vi "acq_and_background.vi"(9 "Acquisition Parameters":refnum<vi>[](array[refnum]), 11 "LightField Automation in":refnum<class "LightField Automation.lvclass">) -> (1 "DAQmx":dbl[][](array[numeric]), 2 "CCD":dbl[](array[numeric]), 3 "LightField Automation out":refnum<class "LightField Automation.lvclass">)   [LabVIEW 2015]
uses:
  lightfield-automation-labview/LightField Automation.lvclass
panel:
  out "Increment piezo":dbl
  out "Piezo":dbl
  out "DAQmx Task Shutter":refnum<k21>
  out "Shutter":string
  out "Background":string
  out "Accumulations":i32
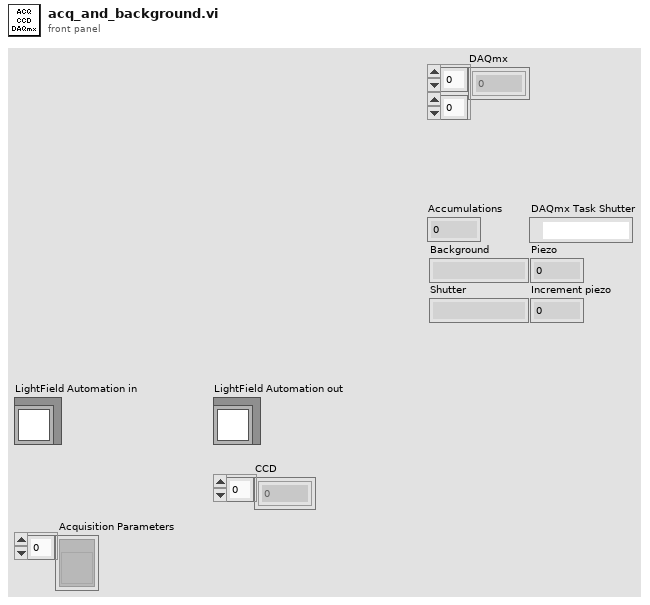
[diagram p1: front panel]
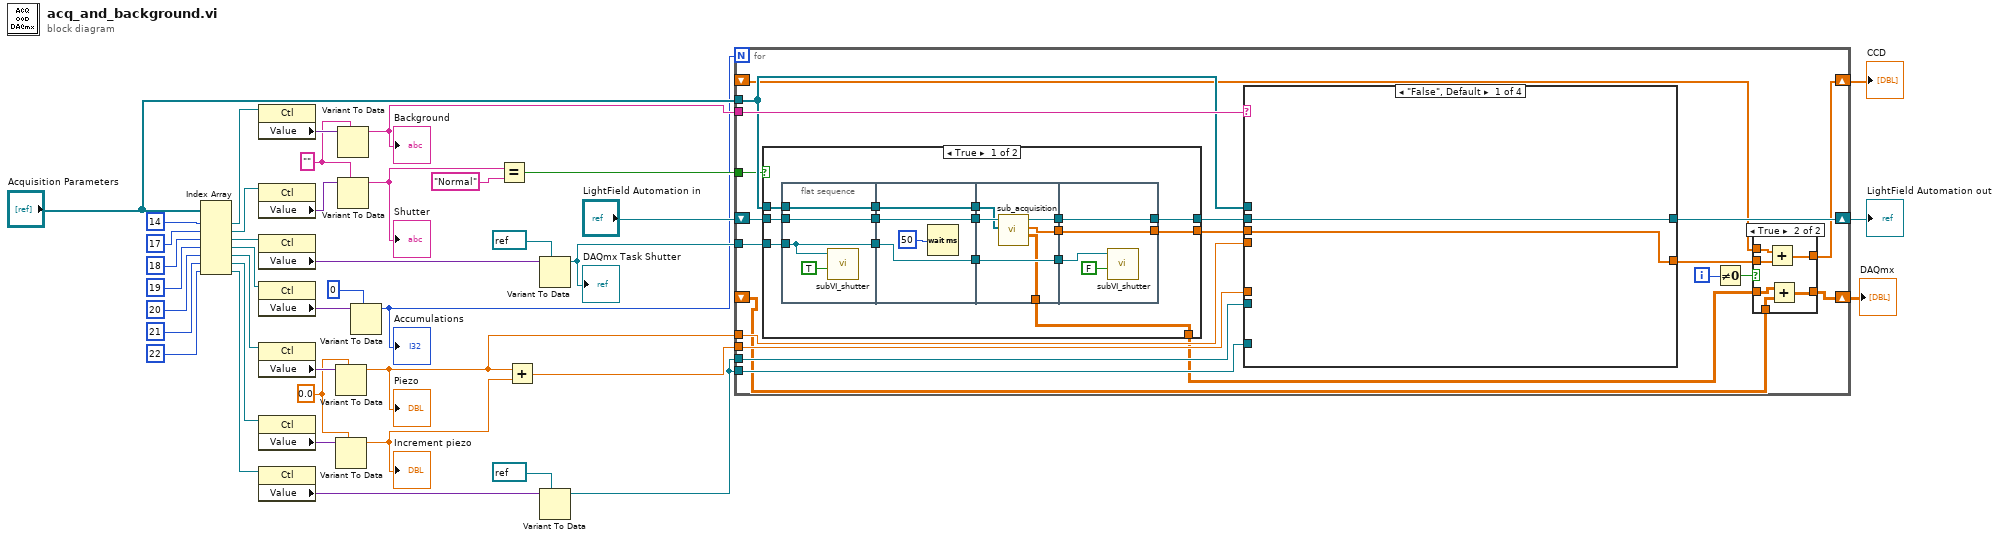
[diagram p0: block diagram]
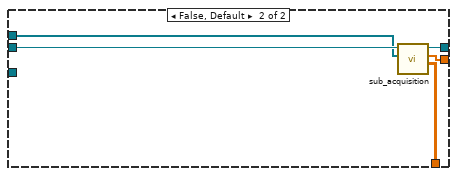
[diagram p3: hidden frame]
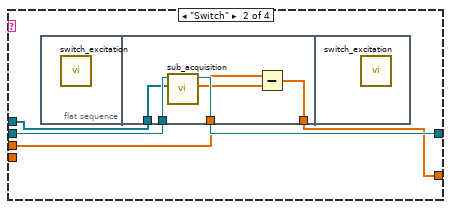
[diagram p4: hidden frame]
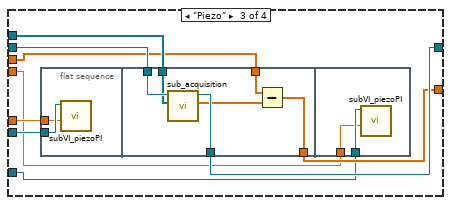
[diagram p5: hidden frame]
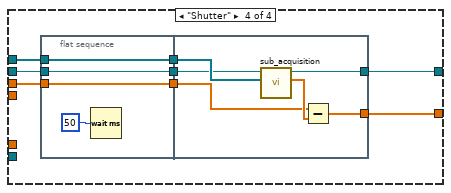
[diagram p6: hidden frame]
diagram:
  w10 = 0.0
  w31 = ""
  n1 = Index Array(array="Acquisition Parameters", index #1=14 ("index"), index #2=17 ("index"), index #3=18, index #4=19 ("index"), index #5=20 ("index"), index #6=21 ("index"), index #7=22 ("index")) -> (element #1=w38:refnum<vi>, element #2=w27:refnum<vi>, element #3=w26:refnum<vi>, element #4=w20:refnum<vi>, element #5=w12:refnum<vi>, element #6=w11:refnum<vi>, element #7=w6:refnum<vi>)
  n2 = property class="Ctl"(reference=w38) -> ("Value"=w37:variant)  [unwired: 1 in, 2 out]
  n3 = property class="Ctl"(reference=w27) -> ("Value"=w35:variant)  [unwired: 1 in, 2 out]
  n4 = property class="Ctl"(reference=w26) -> ("Value"=w25:variant)  [unwired: 1 in, 2 out]
  n5 = property class="Ctl"(reference=w20) -> ("Value"=w21:variant)  [unwired: 1 in, 2 out]
  n6 = property class="Ctl"(reference=w12) -> ("Value"=w14:variant)  [unwired: 1 in, 2 out]
  n7 = property class="Ctl"(reference=w11) -> ("Value"=w13:variant)  [unwired: 1 in, 2 out]
  n8 = property class="Ctl"(reference=w6) -> ("Value"=w8:variant)  [unwired: 1 in, 2 out]
  n9 = Variant To Data(type=w10, Variant=w14) -> (data=w2:dbl)  [unwired: 1 in, 1 out]
  "Piezo" <- w2
  n10 = Variant To Data(type=w10, Variant=w13) -> (data=w4:dbl)  [unwired: 1 in, 1 out]
  "Increment piezo" <- w4
  n11 = Variant To Data(type=w31, Variant=w37) -> (data=w36:string)  [unwired: 1 in, 1 out]
  "Background" <- w36
  n12 = Variant To Data(type=w31, Variant=w35) -> (data=w33:string)  [unwired: 1 in, 1 out]
  "Shutter" <- w33
  n13 = Variant To Data(type=0, Variant=w21) -> (data=w18:i32)  [unwired: 1 in, 1 out]
  "Accumulations" <- w18
  n14 = Equal?(x=w33, y="Normal") -> (x = y?=w30:bool)
  n15 = Add(x=w2, y=w4) -> (x+y=w3:dbl)
  n16 = Variant To Data(type=refnum<k21> refnum ("task out"), Variant=w25) -> (data=w23:refnum<k21>)  [unwired: 1 in, 1 out]
  "DAQmx Task Shutter" <- w23
  n17 = Variant To Data(type=refnum<k21> refnum ("task out"), Variant=w8) -> (data=w5:refnum<k21>)  [unwired: 1 in, 1 out]
  n18 = for {
    N: w18 -> [_]
    tunnel: w36 -> [w57]
    tunnel: "Acquisition Parameters" -> [w56]
    tunnel: w30 -> [w55]
    tunnel: w23 -> [w54]
    shift-right: [w60] -> w41
    shift-left: "LightField Automation in" -> [w58]
    shift-right: [w47] -> w17
    shift-left: _ -> [w49]
    tunnel: w5 -> [w53]
    tunnel: w5 -> [w52]
    tunnel: w3 -> [w51]
    tunnel: w2 -> [w50]
    shift-right: [w43] -> w1
    shift-left: _ -> [w42]
    i -> [w46]
    n19 = case shown="True" w55 {
      tunnel: [w84 w107] -> w61
      tunnel: [w83 w106] -> w59
      tunnel: w58 -> [w82 w105]
      tunnel: w56 -> [w81 w104]
      tunnel: w54 -> [w78 _]
      tunnel: [w70 w103] -> w44
      frame True {
        n20 = flat-sequence {
          tunnel: w81 -> [w87]
          tunnel: w82 -> [w88]
          tunnel: [w88] -> w76
          tunnel: [w87] -> w74
          tunnel: w78 -> [w85]
          tunnel: [w85] -> w72
          tunnel: w76 -> [w92]
          tunnel: [w92] -> w75
          tunnel: w74 -> [w91]
          tunnel: [w91] -> w73
          tunnel: w72 -> [w90]
          tunnel: [w90] -> w71
          tunnel: w75 -> [w96]
          tunnel: w73 -> [w95]
          tunnel: [w98] -> w80
          tunnel: [w97] -> w79
          tunnel: [w94] -> w77
          tunnel: w71 -> [w94]
          tunnel: [w93] -> w70
          tunnel: [w101] -> w83
          tunnel: [w102] -> w84
          tunnel: w80 -> [w102]
          tunnel: w79 -> [w101]
          tunnel: w77 -> [w99]
          frame #0 {
            n21 = call "subVI_shutter.vi"("Shutter"=TRUE, "task out"=w85) -> ()  [unwired: 9 in, 1 out]
          }
          frame #1 {
            n22 = Wait (ms)(milliseconds to wait=u32 50) -> ()  [unwired: 1 out]
          }
          frame #2 {
            n23 = call "sub_acquisition.vi"("LightField Automation in"=w96, "Acquisition Parameters 2"=w95) -> ("LightField Automation out"=w97:refnum<class "LightField Automation.lvclass">, "CCD"=w98:dbl[], "DAQmx"=w93:dbl[][])  [unwired: 5 in, 1 out]
          }
          frame #3 {
            n24 = call "subVI_shutter.vi"("Shutter"=FALSE, "task out"=w99) -> ()  [unwired: 9 in, 1 out]
          }
        }
      }
      frame False, Default {
        n25 = call "sub_acquisition.vi"("LightField Automation in"=w105, "Acquisition Parameters 2"=w104) -> ("LightField Automation out"=w106:refnum<class "LightField Automation.lvclass">, "CCD"=w107:dbl[], "DAQmx"=w103:dbl[][])  [unwired: 5 in, 1 out]
      }
    }
    n26 = case shown="\"False\", Default" w57 {
      tunnel: w59 -> [w109 w114 w129 w145]
      tunnel: [w109 w113 w128 w144] -> w60
      tunnel: w56 -> [_ w112 w127 w146]
      tunnel: w61 -> [w108 w111 w126 w147]
      tunnel: [w108 w110 w125 w143] -> w48
      tunnel: w53 -> [_ _ w124 _]
      tunnel: w52 -> [_ _ w123 _]
      tunnel: w51 -> [_ _ w122 _]
      tunnel: w50 -> [_ _ w121 _]
      frame "False", Default {
      }
      frame "Switch" {
        n27 = flat-sequence {
          tunnel: w114 -> [w120]
          tunnel: [w119] -> w113
          tunnel: w112 -> [w118]
          tunnel: w111 -> [w116]
          tunnel: [w115] -> w110
          frame #0 {
            n28 = call "switch_excitation.vi"() -> ()  [unwired: 2 in, 2 out]
          }
          frame #1 {
            n29 = call "sub_acquisition.vi"("LightField Automation in"=w120, "Acquisition Parameters 2"=w118) -> ("LightField Automation out"=w119:refnum<class "LightField Automation.lvclass">, "CCD"=w117:dbl[])  [unwired: 5 in, 2 out]
            n30 = Subtract(x=w116, y=w117) -> (x-y=w115:dbl[])
          }
          frame #2 {
            n31 = call "switch_excitation.vi"() -> ()  [unwired: 2 in, 2 out]
          }
        }
      }
      frame "Piezo" {
        n32 = flat-sequence {
          tunnel: w124 -> [w131]
          tunnel: w122 -> [w130]
          tunnel: w129 -> [w137]
          tunnel: [w136] -> w128
          tunnel: w127 -> [w135]
          tunnel: w126 -> [w133]
          tunnel: [w132] -> w125
          tunnel: w123 -> [w139]
          tunnel: w121 -> [w138]
          frame #0 {
            n33 = call "subVI_piezoPI.vi"("data"=w130, "task/channels in"=w131) -> ()  [unwired: 9 in, 1 out]
          }
          frame #1 {
            n34 = call "sub_acquisition.vi"("LightField Automation in"=w137, "Acquisition Parameters 2"=w135) -> ("LightField Automation out"=w136:refnum<class "LightField Automation.lvclass">, "CCD"=w134:dbl[])  [unwired: 5 in, 2 out]
            n35 = Subtract(x=w133, y=w134) -> (x-y=w132:dbl[])
          }
          frame #2 {
            n36 = call "subVI_piezoPI.vi"("data"=w138, "task/channels in"=w139) -> ()  [unwired: 9 in, 1 out]
          }
        }
      }
      frame "Shutter" {
        n37 = flat-sequence {
          tunnel: w145 -> [w149]
          tunnel: w146 -> [w150]
          tunnel: w147 -> [w151]
          tunnel: [w151] -> w142
          tunnel: [w150] -> w141
          tunnel: [w149] -> w140
          tunnel: [w153] -> w144
          tunnel: [w152] -> w143
          tunnel: w142 -> [w156]
          tunnel: w141 -> [w155]
          tunnel: w140 -> [w154]
          frame #0 {
            n38 = Wait (ms)(milliseconds to wait=u32 50) -> ()  [unwired: 1 out]
          }
          frame #1 {
            n39 = call "sub_acquisition.vi"("LightField Automation in"=w154, "Acquisition Parameters 2"=w155) -> ("LightField Automation out"=w153:refnum<class "LightField Automation.lvclass">, "CCD"=w157:dbl[])  [unwired: 5 in, 2 out]
            n40 = Subtract(x=w156, y=w157) -> (x-y=w152:dbl[])
          }
        }
      }
    }
    n41 = Not Equal To 0?(x=w46) -> (x != 0?=w45:bool)
    n42 = case shown="True" w45 {
      tunnel: w49 -> [_ w69]
      tunnel: w48 -> [w63 w68]
      tunnel: [w63 w67] -> w47
      tunnel: w44 -> [w62 w66]
      tunnel: [w62 w64] -> w43
      tunnel: w42 -> [_ w65]
      frame False {
      }
      frame True {
        n43 = Add(x=w69, y=w68) -> (x+y=w67:dbl[])
        n44 = Add(x=w66, y=w65) -> (x+y=w64:dbl[][])
      }
    }
  }
  "CCD" <- w17
  "LightField Automation out" <- w41
  "DAQmx" <- w1
